vi "createState.vi"(8 "error in (no error)":errorcluster, 10 "State:":T1, 11 "StateFactory in":refnum<class "StateFactory.lvclass">) -> (0 "error out":errorcluster, 2 "State.lvclass":refnum<class "State.lvclass">, 3 "StateFactory out":refnum<class "StateFactory.lvclass">)   [LabVIEW 2015, in "StateFactory.lvclass"]
uses:
  StateFactory.lvclass
  Typedefs/StateSelector.ctl
  State/State.lvclass
  States/FaultState/FaultState.lvclass
  States/OffState/OffState.lvclass
  States/StandbyState/StandbyState.lvclass
  States/StoppedState/StoppedState.lvclass
  States/WaitingForSettledPState/WaitingForSettledPState.lvclass
  States/WaitingForSettledSTState/WaitingForSettledSTState.lvclass
  States/RampingUpPressurePState/RampingUpPressurePState.lvclass
  States/RampingUpPressureSTState/RampingUpPressureSTState.lvclass
  Typedefs/M1M3SSSTypedefs.lvlib
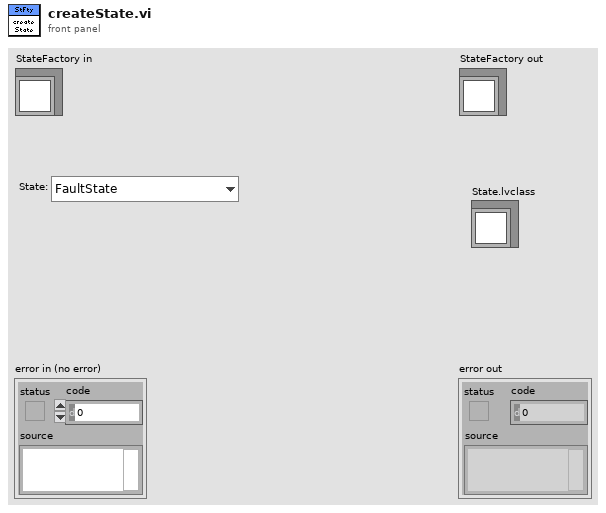
[diagram p1: front panel]
types:
  T1 = typedef "M1M3SSSTypedefs.lvlib/StateSelector.ctl" = enum16{"FaultState", "OffState", "RampingUpPressurePState", "RampingUpPressureSTState", "StandbyState", "StoppedState", "WaitingForSettledPState", "WaitingForSettledSTState"}
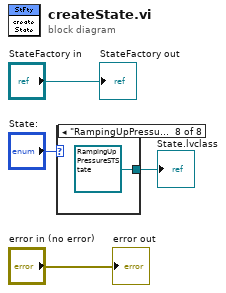
[diagram p0: block diagram]
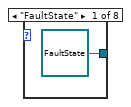
[diagram p2: hidden frame]
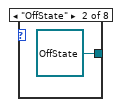
[diagram p3: hidden frame]
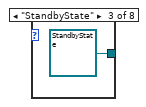
[diagram p4: hidden frame]
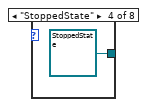
[diagram p5: hidden frame]
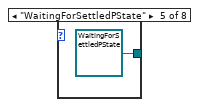
[diagram p6: hidden frame]
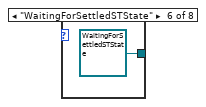
[diagram p7: hidden frame]
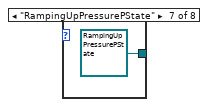
[diagram p8: hidden frame]
diagram:
  n1 = case shown="\"RampingUpPressureSTState\"" "State:" {
    tunnel: [refnum<class "FaultState.lvclass"> refnum ("FaultState.lvclass") refnum<class "OffState.lvclass"> refnum ("ShutdownState.lvclass") refnum<class "StandbyState.lvclass"> refnum ("StandbyState.lvclass") refnum<class "StoppedState.lvclass"> refnum ("StoppedState.lvclass") refnum<class "WaitingForSettledPState.lvclass"> refnum ("WaitingForSettledPState.lvclass") refnum<class "WaitingForSettledSTState.lvclass"> refnum ("WaitingForSettledSTState.lvclass") refnum<class "RampingUpPressurePState.lvclass"> refnum ("RampingUpPressurePState.lvclass") refnum<class "RampingUpPressureSTState.lvclass"> refnum ("RampingUpPressureSTState.lvclass")] -> w1
    frame "FaultState" {
    }
    frame "OffState" {
    }
    frame "StandbyState" {
    }
    frame "StoppedState" {
    }
    frame "WaitingForSettledPState" {
    }
    frame "WaitingForSettledSTState" {
    }
    frame "RampingUpPressurePState" {
    }
    frame "RampingUpPressureSTState" {
    }
  }
  "State.lvclass" <- w1
  "error out" <- "error in (no error)"
  "StateFactory out" <- "StateFactory in"
